vi "Bin XYZ Data.vi"(8 "label":string, 9 "y data":dbl[](array[numeric]), 10 "x data":dbl[](array[numeric]), 11 "z data":dbl[](array[numeric])) -> (2 "z labels":string[](array[string]), 3 "z curves":cluster{dbl[], dbl[]}[](array[cluster]))   [LabVIEW 2020]
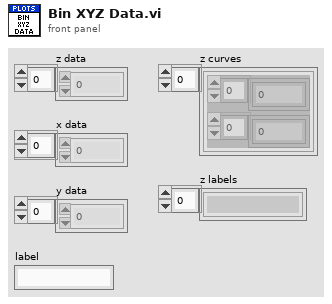
[diagram p1: front panel]
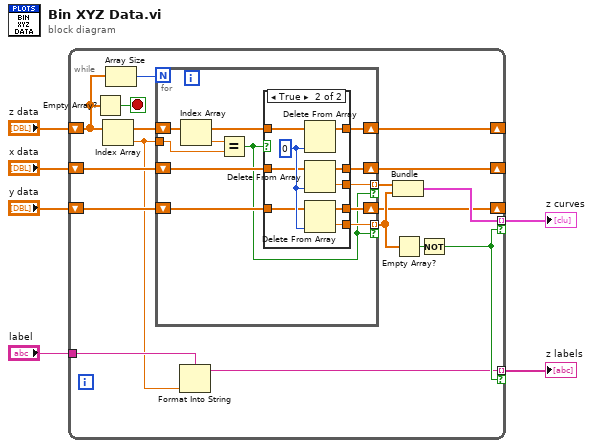
[diagram p0: block diagram]
diagram:
  n1 = while {
    tunnel: "label" -> [w9]
    tunnel: [w7] -> w6 mode=indexing if=w17
    tunnel: [w19] -> w5 mode=indexing if=w17
    shift-right: [w12] -> _
    shift-left: "z data" -> [w13]
    shift-right: [w11] -> _
    shift-left: "x data" -> [w21]
    shift-right: [w10] -> _
    shift-left: "y data" -> [w20]
    stop <- w22 stop-if-true
    n2 = Empty Array?(array=w13) -> (empty?=w22:bool)
    n3 = Index Array(array=w13) -> (element=w8:dbl)  [unwired: 1 in]
    n4 = Array Size(array=w13) -> (size(s)=w14:i32)
    n5 = for {
      N: w14 -> [_]
      shift-right: [w31] -> w12
      shift-left: w13 -> [w33]
      tunnel: w8 -> [w30]
      shift-right: [w27] -> w11
      shift-left: w21 -> [w29]
      shift-right: [w26] -> w10
      shift-left: w20 -> [w28]
      tunnel: [w25] -> w15 mode=indexing if=w23
      tunnel: [w24] -> w16 mode=indexing if=w23
      n6 = Index Array(array=w33) -> (element=w32:dbl)  [unwired: 1 in]
      n7 = Equal?(x=w32, y=w30) -> (x = y?=w23:bool)
      n8 = case shown="True" w23 {
        tunnel: w33 -> [w36 w45]
        tunnel: [w36 w44] -> w31
        tunnel: w29 -> [w35 w42]
        tunnel: w28 -> [w34 w41]
        tunnel: [w35 w40] -> w27
        tunnel: [w34 w39] -> w26
        tunnel: [_ w38] -> w25
        tunnel: [_ w37] -> w24
        frame False {
        }
        frame True {
          w43 = 0 ("index")
          n9 = Delete From Array(array=w45, index=w43) -> (array with subset deleted=w44:dbl[])  [unwired: 1 in, 1 out]
          n10 = Delete From Array(array=w42, index=w43) -> (deleted portion=w37:dbl, array with subset deleted=w40:dbl[])  [unwired: 1 in]
          n11 = Delete From Array(array=w41, index=w43) -> (deleted portion=w38:dbl, array with subset deleted=w39:dbl[])  [unwired: 1 in]
        }
      }
    }
    n12 = Format Into String(format string=w9, w8) -> (resulting string=w7:string)  [unwired: 2 in, 1 out]
    n13 = Bundle(w16, w15) -> (w19:cluster{dbl[], dbl[]})  [unwired: 1 in]
    n14 = Empty Array?(array=w15) -> (empty?=w18:bool)
    n15 = Not(x=w18) -> (.not. x?=w17:bool)
  }
  "z labels" <- w6
  "z curves" <- w5
